vi "Year2016_Question4.vi"() -> ()   [LabVIEW 2015]
panel:
  in  "stop":bool
  out "Waveform Chart":cluster{dbl, dbl}(graph)
  in  "phi2":dbl
  in  "omega2":dbl
  in  "A2":dbl
  in  "phi1":dbl
  in  "omega1":dbl
  in  "A1":dbl
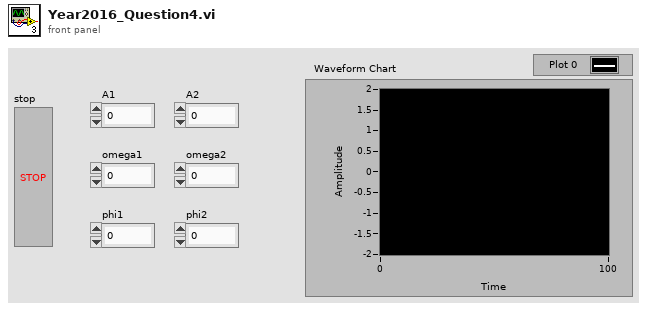
[diagram p1: front panel]
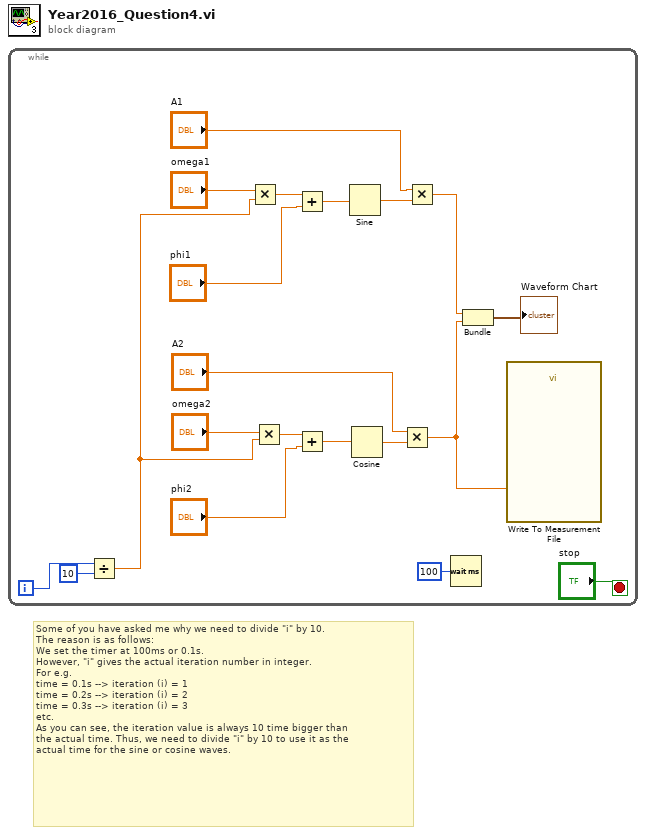
[diagram p0: block diagram]
diagram:
  # "Some of you have asked me why we need to divide \"i\" by 10.\nThe reason is as follows:\nWe set the timer at 100ms or 0.1s.\nHowever, \"i\" gives the actual iteration number in integer.\nFor e.g.\ntime = 0.1s --> iteration (i) = 1\ntime = 0.2s --> iteration (i) = 2\ntime = 0.3s --> iteration (i) = 3\netc.\nAs you can see, the iteration value is always 10 time bigger than \nthe actual time. Thus, we need to divide \"i\" by 10 to use it as the\nactual time for the sine or cosine waves."
  n1 = while {
    i -> [w19]
    stop <- "stop" stop-if-true
    n2 = Divide(x=w19, y=10) -> (x/y=w16:dbl)
    n3 = Multiply(x="omega1", y=w16) -> (x*y=w14:dbl)
    n4 = Multiply(x="omega2", y=w16) -> (x*y=w12:dbl)
    n5 = Add(x=w14, y="phi1") -> (x+y=w10:dbl)
    n6 = Add(x=w12, y="phi2") -> (x+y=w9:dbl)
    n7 = Sine(x=w10) -> (sin(x)=w7:dbl)
    n8 = Cosine(x=w9) -> (cos(x)=w5:dbl)
    n9 = Multiply(x="A2", y=w5) -> (x*y=w1:dbl)
    n10 = Multiply(x="A1", y=w7) -> (x*y=w3:dbl)
    n11 = Wait (ms)(milliseconds to wait=u32 100) -> ()  [unwired: 1 out]
    n12 = Bundle(w3, w1) -> (→"Waveform Chart":cluster{dbl, dbl})  [unwired: 1 in]
    n13 = call "Write To Measurement File"("Signals"=w1) -> ()  [unwired: 16 in, 3 out]
  }
